vi "lineVariance.vi"(10 "Line":cluster{"X":dbl, "Y":dbl}[](array[cluster])) -> (2 "lineAngle":dbl)   [LabVIEW 2016]
uses:
  <vilib>/Analysis/6fits.llb/Curve Fitting Criteria.ctl
  <vilib>/Analysis/NI_AALPro.lvlib
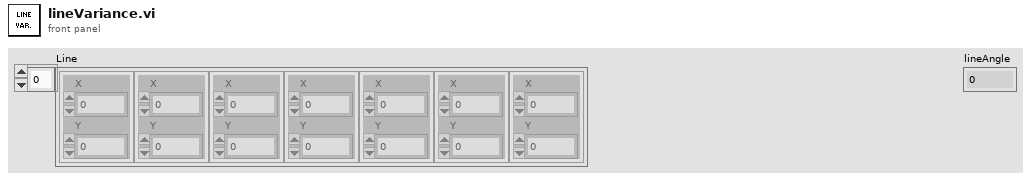
[diagram p1: front panel]
types:
  T1 = cluster{"slope min":dbl, "slope max":dbl, "intercept min":dbl, "intercept max":dbl}
  T2 = typedef "NI_AALPro.lvlib/Curve Fitting Criteria.ctl" = u16
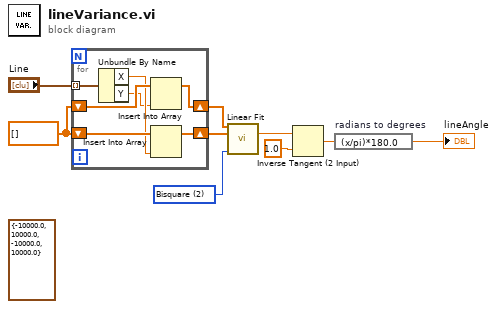
[diagram p0: block diagram]
diagram:
  (unwired) T1 {"slope min"=-10000.0, "slope max"=10000.0, "intercept min"=-10000.0, "intercept max"=10000.0} ("parameter bounds")
  w7 = T2 2 items=["Least Square", "Least Absolute Residual", "Bisquare"] ("method")
  w8 = dbl[] []
  n1 = for {
    tunnel: "Line" -> [w16] mode=indexing
    shift-right: [w14] -> w1
    shift-left: w8 -> [w13]
    shift-right: [w15] -> w2
    shift-left: w8 -> [w12]
    n2 = Unbundle By Name(w16) -> ("X"=w11:dbl, "Y"=w10:dbl)
    n3 = Insert Into Array(array=w13, new element=w10) -> (w14:dbl[])  [unwired: 1 in]
    n4 = Insert Into Array(array=w12, new element=w11) -> (w15:dbl[])  [unwired: 1 in]
  }
  n5 = call <vilib>:"Linear Fit.vi"("Y"=w1, "X"=w2, "method"=w7) -> ("slope"=w3:dbl)  [unwired: 8 in, 4 out]
  n6 = Inverse Tangent (2 Input)(1:1.0 ("x"), 2:w3) -> (0:w5:dbl)
  n7 = expression code="(x/pi)*180.0" "radians to degrees"(w5) -> (→"lineAngle":dbl)
